vi "5V-Test.vi"() -> ()   [LabVIEW 2010]
uses:
  <vilib>/eio/EIONode/EIONode.xnode
panel:
  in  "Mod6/DIO21":bool
  out "Mod1/AI30":fxp<+/-,26,5> format="%.23g"
  in  "stop":bool
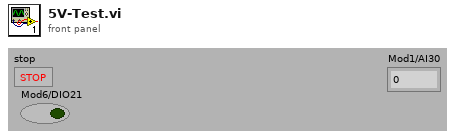
[diagram p1: front panel]
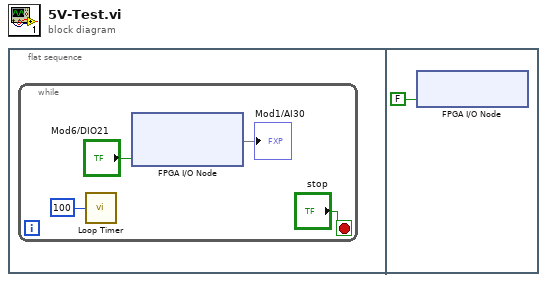
[diagram p0: block diagram]
diagram:
  n1 = flat-sequence {
    frame #0 {
      n2 = while {
        stop <- "stop" stop-if-true
        n3 = call "Loop Timer"("Count(mSec)"=u32 100) -> ()  [unwired: 1 out]
        n4 = xnode "FPGA I/O Node"("Mod6/DIO21"="Mod6/DIO21") -> ("Mod1/AI30"=→"Mod1/AI30")  [unwired: 2 in, 2 out]
      }
    }
    frame #1 {
      n5 = xnode "FPGA I/O Node"("Mod6/DIO21"=FALSE) -> ()  [unwired: 1 in, 1 out]
    }
  }
